vi "Global Configuration File Access.vi"(7 "Command":T1, 8 "error in":errorcluster, 10 "configuration file path":path, 11 "EMS Generic in":refnum<class "EMS Generic.lvclass">) -> (0 "error out":errorcluster, 3 "EMS Generic out":refnum<class "EMS Generic.lvclass">)   [LabVIEW 2018, in "EMS Generic Actor.lvlib" / "EMS Generic.lvclass"]
uses:
  EMS Generic.lvclass
  EMS User Interface Actor/EMS User Interface/Controls/Configuration/File Access Command.ctl
  EMS Generic.lvclass/EMS Generic.ctl
  Controls/Global Configuration.ctl
  <vilib>/ORNL/CSEISMIC DDS/CSEISMIC DDS Base/Data Types/Controls/DeviceID.ctl
  <vilib>/Utility/config.llb/NI_LVConfig.lvlib
  <vilib>/ORNL/CSEISMIC DDS/CSEISMIC DDS Base/CSEISMIC DDS.lvclass
  Utilities/Status Messaging.llb/Status Messaging.lvlib
  EMS User Interface Actor/EMS User Interface/EMS User Interface.lvclass
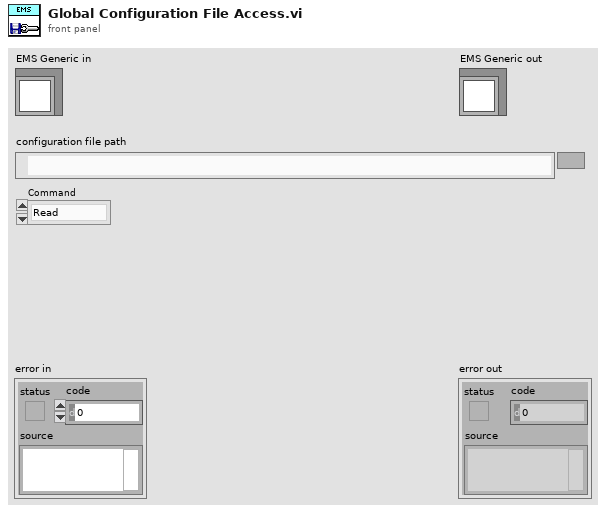
[diagram p1: front panel]
types:
  T1 = typedef "EMS User Interface Actor.lvlib/EMS User Interface.lvclass/File Access Command.ctl" = enum16{"Read", "Write"}
  T2 = typedef "NI_LVConfig.lvlib/Config Data RefNum.ctl" = refnum<k1>
  T3 = typedef "EMS Generic Actor.lvlib/EMS Generic.lvclass/Global Configuration.ctl" = cluster{"Microgrid ID":u8, "VF Device ID":T4, "Ongrid VF Priority":T4[], "Offgrid VF Priority":T4[], "AutoSwap Offgrid VF":u32, "AutoSwap Offgrid VF Delay (sec)":dbl, "AutoSwap Resynch VF":u32, "PCC Device ID":T4, "Device ID Array":T4[], "Nominal Voltage":dbl, "Nominal Frequency":dbl, "Resynch Timeout (sec)":dbl, "Island VF Activate Timeout (sec)":dbl, "Island PCC Target Power (kW)":dbl, "Island PCC Target Power Timeout (sec)":dbl, "Island Grid Settle Time (sec)":dbl, "Island PCC Failure Timeout (sec)":dbl, "Activation Devices Present Timeout (sec)":dbl, "Activation Devices Activated Timeout (sec)":dbl, "Blackstart VF GenMode Wait (sec)":dbl, "Blackstart VF DERCtrl Wait (sec)":dbl, "Blackstart Success Wait (sec)":dbl, "OnGrid Optimization Delay (sec)":dbl, "OffGrid Optimization Delay (sec)":dbl, "Resynch Frequency (Hz)":dbl, "Optimization Path":string}
  T4 = typedef "CSEISMIC DDS.lvlib/CSEISMIC DDS.lvclass/DeviceID.ctl" = string
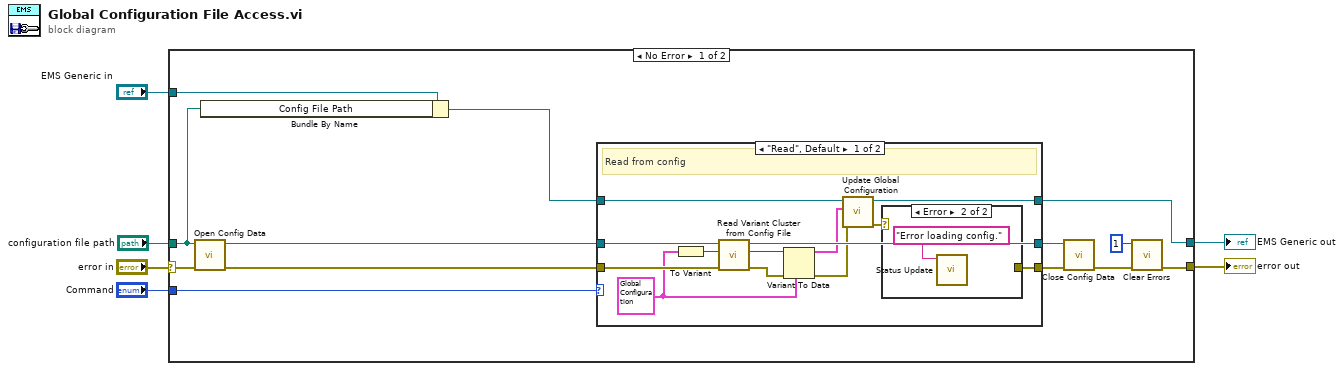
[diagram p0: block diagram]
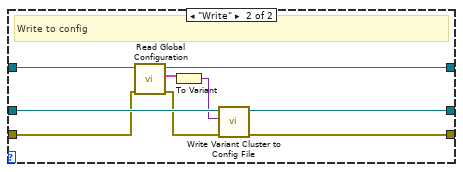
[diagram p3: hidden frame]
diagram:
  n1 = case shown="No Error" "error in" {
    selector: "error in" -> [w19 w45]
    tunnel: [w8 w45] -> w5
    tunnel: [w9 w44] -> w3
    tunnel: "EMS Generic in" -> [w13 w44]
    tunnel: "Command" -> [w15 _]
    tunnel: "configuration file path" -> [w14 _]
    frame No Error {
      n2 = call <vilib>:"Open Config Data.vi"("error in (no error)"=w19, "configuration file path"=w14) -> ("error out"=w12:errorcluster, "refnum"=w18:T2)  [unwired: 7 in, 1 out]
      n3 = Bundle By Name(cluster=w13, "Config File Path"=w14) -> (w10:refnum<class "EMS Generic.lvclass">)
      n4 = case shown="\"Read\", Default" w15 {
        tunnel: w18 -> [w32 w43]
        tunnel: w12 -> [w30 w37]
        tunnel: [w20 w42] -> w16
        tunnel: [w31 w41] -> w17
        tunnel: w10 -> [w25 w40]
        tunnel: [w24 w35] -> w9
        frame "Read", Default {
          w26 = T3 {"Microgrid ID"=1, "VF Device ID"="", "Ongrid VF Priority"=[], "Offgrid VF Priority"=[], "AutoSwap Offgrid VF"=0, "AutoSwap Offgrid VF Delay (sec)"=0.0, "AutoSwap Resynch VF"=0, "PCC Device ID"="", "Device ID Array"=[], "Nominal Voltage"=0.0, "Nominal Frequency"=0.0, "Resynch Timeout (sec)"=0.0, "Island VF Activate Timeout (sec)"=90.0, "Island PCC Target Power (kW)"=0.0, "Island PCC Target Power Timeout (sec)"=0.0, "Island Grid Settle Time (sec)"=0.0, "Island PCC Failure Timeout (sec)"=0.0, "Activation Devices Present Timeout (sec)"=0.0, "Activation Devices Activated Timeout (sec)"=0.0, "Blackstart VF GenMode Wait (sec)"=0.0, "Blackstart VF DERCtrl Wait (sec)"=0.0, "Blackstart Success Wait (sec)"=0.0, "OnGrid Optimization Delay (sec)"=0.0, "OffGrid Optimization Delay (sec)"=0.0, "Resynch Frequency (Hz)"=0.0, "Optimization Path"=""} ("Global Configuration")
          # "Read from config"
          n5 = To Variant(anything=w26) -> (Variant=w27:variant)
          n6 = call "Read Variant Cluster from Config File.vi"("error in"=w30, "Variant Cluster in"=w27, "Config Refnum in"=w32) -> ("error out"=w29:errorcluster, "Variant Cluster out"=w28:variant, "Config Refnum out"=w31:T2)  [unwired: 5 in, 1 out]
          n7 = Variant To Data(error in=w29, type=w26, Variant=w28) -> (data=w23:T3, error out=w22:errorcluster)
          n8 = call "Update Global Configuration.vi"("error in (no error)"=w22, "Global Configuration"=w23, "EMS Generic in"=w25) -> ("error out"=w21:errorcluster, "EMS Generic out"=w24:refnum<class "EMS Generic.lvclass">)  [unwired: 7 in]
          n9 = case shown="Error" w21 {
            selector: w21 -> [w33 _]
            tunnel: [w33 _] -> w20
            frame No Error {
            }
            frame Error {
              n10 = call "Status Update.vi"("Status Update"="Error loading config.") -> ()  [unwired: 9 in, 2 out]
            }
          }
        }
        frame "Write" {
          # "Write to config"
          n11 = call "Read Global Configuration.vi"("error in"=w37, "EMS Generic in"=w40) -> ("error out"=w36:errorcluster, "Global Configuration"=w39:T3, "dup EMS Generic out"=w35:refnum<class "EMS Generic.lvclass">)  [unwired: 7 in]
          n12 = To Variant(anything=w39) -> (Variant=w38:variant)
          n13 = call "Write Variant Cluster to Config File.vi"("error in"=w36, "Variant Configuration Object"=w38, "Config Refnum in"=w43) -> ("error out"=w42:errorcluster, "Config Refnum out"=w41:T2)  [unwired: 7 in]
        }
      }
      n14 = call <vilib>:"Close Config Data.vi"("error in (no error)"=w16, "refnum"=w17) -> ("error out"=w11:errorcluster)  [unwired: 8 in, 1 out]
      n15 = call <vilib>:"Clear Errors.vi"("error in (no error)"=w11, "specific error code to clear (0: all)"=1) -> ("error out"=w8:errorcluster)  [unwired: 4 in, 1 out]
    }
    frame Error {
    }
  }
  "error out" <- w5
  "EMS Generic out" <- w3
